vi "Test Read InteropAssembly.vi"() -> ()   [LabVIEW 2020]
uses:
  C:/Users/dzoni/Documents/NJ/Playground/LV/TCP Client/client/builds/ClientApp1/ClientApp1.dll
  builds/ClientApp1/ClientApp1.dll
panel:
  in  "Constructor Selection":T1(ring)=enum."Constructor Ptr"
  out "Size":i32
  out "Size 1":i32
  out "IsValid":bool
  out "ID":string
  out "Port":u16
  out "Data 2":string
  out "Data":string
  out "Address":string
  out "error out":errorcluster
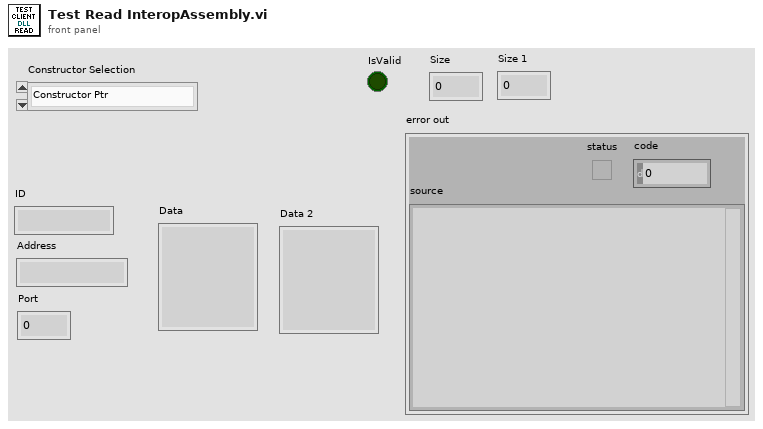
[diagram p1: front panel]
types:
  T1 = enum16{"No Constructor", "Constructor new", "Constructor Ptr"}
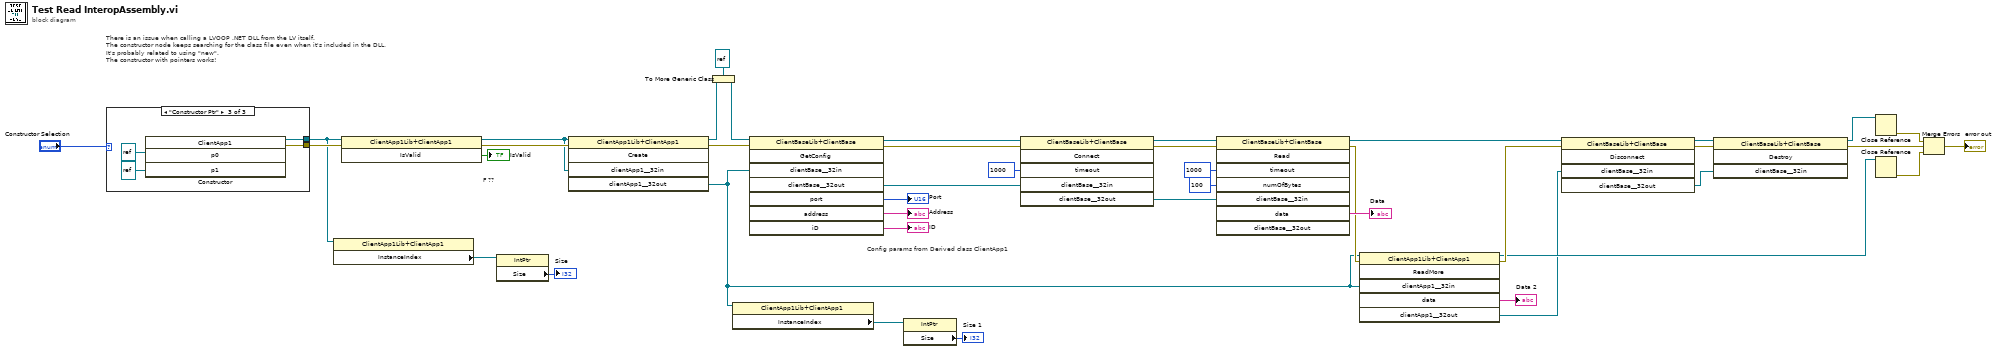
[diagram p0: block diagram]
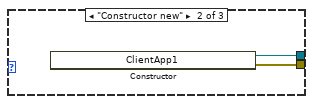
[diagram p3: hidden frame]
diagram:
  # "Config params from Derived class ClientApp1"
  # "F ??"
  # "There is an issue when calling a LVOOP .NET DLL from the LV itself.\nThe constructor node keeps searching for the class file even when it's included in the DLL.\nIt's probably related to using \"new\".\nThe constructor with pointers works!"
  n1 = case shown="\"Constructor Ptr\"" "Constructor Selection" {
    tunnel: [_ w43 w48] -> w10
    tunnel: [_ w44 w47] -> w6
    frame "No Constructor", Default {
    }
    frame "Constructor new" {
      n2 = constructor class="ClientApp1Lib+ClientApp1"() -> (reference out=w44:refnum<k24>, error out=w43:errorcluster)  [unwired: 3 in, 1 out]
    }
    frame "Constructor Ptr" {
      n3 = constructor class="ClientApp1Lib+ClientApp1"("p0"=refnum<k24> refnum, "p1"=refnum<k24> refnum) -> (reference out=w47:refnum<k24>, error out=w48:errorcluster)  [unwired: 3 in, 3 out]
    }
  }
  n4 = property class="ClientApp1Lib+ClientApp1"(reference=w6) -> ("InstanceIndex"=w3:refnum<k24>)  [unwired: 1 in, 2 out]
  n5 = invoke class="ClientApp1Lib+ClientApp1" method="IsValid"(reference=w6, error in=w10) -> (reference out=w8:refnum<k24>, error out=w9:errorcluster, "IsValid"=→"IsValid":bool)  [unwired: 1 in]
  n6 = property class="IntPtr"(reference=w3) -> ("Size"=→"Size":i32)  [unwired: 1 in, 2 out]
  n7 = invoke class="ClientApp1Lib+ClientApp1" method="Create"(reference=w8, error in=w9, "clientApp1__32in"=w8) -> (reference out=w15:refnum<k24>, error out=w42:errorcluster, "clientApp1__32out"=w7:refnum<k24>)  [unwired: 2 in, 2 out]
  n8 = To More Generic Class(target class=refnum<k24> refnum, reference=w15) -> (generic class reference=w14:refnum<k24>)
  n9 = property class="ClientApp1Lib+ClientApp1"(reference=w7) -> ("InstanceIndex"=w5:refnum<k24>)  [unwired: 1 in, 2 out]
  n10 = invoke class="ClientBaseLib+ClientBase" method="GetConfig"(reference=w14, error in=w42, "clientBase__32in"=w7) -> (reference out=w38:refnum<k24>, error out=w36:errorcluster, "clientBase__32out"=w37:refnum<k24>, "port"=→"Port":u16, "address"=→"Address":string, "iD"=→"ID":string)  [unwired: 5 in, 2 out]
  n11 = property class="IntPtr"(reference=w5) -> ("Size"=→"Size 1":i32)  [unwired: 1 in, 2 out]
  n12 = invoke class="ClientBaseLib+ClientBase" method="Connect"(reference=w38, error in=w36, "timeout"=1000, "clientBase__32in"=w37) -> (reference out=w34:refnum<k24>, error out=w33:errorcluster, "clientBase__32out"=w30:refnum<k24>)  [unwired: 2 in, 3 out]
  n13 = invoke class="ClientBaseLib+ClientBase" method="Read"(reference=w34, error in=w33, "timeout"=1000, "numOfBytes"=100, "clientBase__32in"=w30) -> (reference out=w26:refnum<k24>, error out=w28:errorcluster, "data"=→"Data":string)  [unwired: 3 in, 5 out]
  n14 = invoke class="ClientApp1Lib+ClientApp1" method="ReadMore"(reference=w7, error in=w28, "clientApp1__32in"=w7) -> (reference out=w20:refnum<k24>, error out=w25:errorcluster, "data"=→"Data 2":string, "clientApp1__32out"=w12:refnum<k24>)  [unwired: 3 in, 2 out]
  n15 = invoke class="ClientBaseLib+ClientBase" method="Disconnect"(reference=w26, error in=w25, "clientBase__32in"=w12) -> (reference out=w22:refnum<k24>, error out=w23:errorcluster, "clientBase__32out"=w24:refnum<k24>)  [unwired: 2 in, 2 out]
  n16 = invoke class="ClientBaseLib+ClientBase" method="Destroy"(reference=w22, error in=w23, "clientBase__32in"=w24) -> (reference out=w21:refnum<k24>, error out=w19:errorcluster)  [unwired: 1 in, 2 out]
  n17 = Close Reference(reference=w21) -> (error out=w17:errorcluster)  [unwired: 1 in]
  n18 = Close Reference(reference=w20) -> (error out=w16:errorcluster)  [unwired: 1 in]
  n19 = Merge Errors(w17, w19, w16) -> (→"error out":errorcluster)
